vi "PS Control (RT).vi"() -> ()   [LabVIEW 2019]
uses:
  <vilib>/rvi/interface/nirviReadWriteControl/nirviReadWriteControl.xnode
  <vilib>/rvi/interface/Simulation/niFpgaSimulationCallBeginRW.vi
  <vilib>/rvi/errors/niLvFpgaAdjustHostInterfaceError.vi
  <vilib>/addons/control/pid/NI_PID_pid.lvlib
  <vilib>/addons/control/pid/pid.llb/PID (DBL).vi
  <vilib>/rvi/interface/nirviOpenFPGA/nirviOpenFPGA.xnode
  FPGA/bitfiles/PS Control (FPGA).lvbitx
  <vilib>/ptbypt/NI_PtbyPt.lvlib
  <vilib>/Analysis/3filter.llb/Filter Passband Type.ctl
  <vilib>/Analysis/NI_AALBase.lvlib
  <vilib>/FPGAPlugInAG/sbRIO-9626/niLvFpga_Open_sbRIO-9626.vi
  <vilib>/rvi/interface/common/dynamic/niFpgaDynamicAddResources.vi
panel:
  in  "PS4 Remote Control":bool=TRUE
  in  "PS3 Remote Control":bool=TRUE
  in  "PS2 Remote Control":bool=TRUE
  in  "PS1 Remote Control":bool=TRUE
  out "CPU Usage:":dbl=7.74131899555212 format="%.1f"
  in  "Scale 4":dbl=2.0
  in  "Offset 4":dbl
  out "AI 3":fxp<+/-,24,5>
  in  "PS CMD 4":dbl format="%.2f"
  in  "dt (s) 4":dbl=-1.0 format="%.3f"
  in  "PID gains 4":T1={"proportional gain"=1.0, "integral time"=0.01, "derivative time"=0.0} {"derivative time" format="%.3f"; "integral time" format="%.3f"; "proportional gain" format="%.3f"}
  in  "Output Range 4":cluster{"output high":dbl, "output low":dbl}={"output high"=8.0, "output low"=0.0} {"output low" format="%.2f"; "output high" format="%.2f"}
  out "PS Feedback 4":dbl format="%0.2f"
  out "AO 3":fxp<+/-,20,5>
  in  "Scale 3":dbl=2.0
  in  "Offset 3":dbl
  out "AI 2":fxp<+/-,24,5>
  in  "PS CMD 3":dbl format="%.2f"
  in  "dt (s) 3":dbl=-1.0 format="%.3f"
  in  "PID gains 3":T1={"proportional gain"=1.0, "integral time"=0.01, "derivative time"=0.0} {"derivative time" format="%.3f"; "integral time" format="%.3f"; "proportional gain" format="%.3f"}
  in  "Output Range 3":cluster{"output high":dbl, "output low":dbl}={"output high"=8.0, "output low"=0.0} {"output low" format="%.2f"; "output high" format="%.2f"}
  out "PS Feedback 3":dbl format="%0.2f"
  out "AO 2":fxp<+/-,20,5>
  in  "Scale 2":dbl=2.0
  in  "Offset 2":dbl
  out "AI 1":fxp<+/-,24,5>
  in  "PS CMD 2":dbl format="%.2f"
  in  "dt (s) 2":dbl=-1.0 format="%.3f"
  in  "PID gains 2":T1={"proportional gain"=1.0, "integral time"=0.01, "derivative time"=0.0} {"derivative time" format="%.3f"; "integral time" format="%.3f"; "proportional gain" format="%.3f"}
  in  "Output Range 2":cluster{"output high":dbl, "output low":dbl}={"output high"=8.0, "output low"=0.0} {"output low" format="%.2f"; "output high" format="%.2f"}
  out "PS Feedback 2":dbl format="%0.2f"
  out "AO 1":fxp<+/-,20,5>
  in  "Loop Timer (uSec)":u32=10000
  out "AO 0":fxp<+/-,20,5>
  out "PS Feedback 1":dbl format="%0.2f"
  in  "Output Range 1":cluster{"output high":dbl, "output low":dbl}={"output high"=8.0, "output low"=0.0} {"output low" format="%.2f"; "output high" format="%.2f"}
  in  "PID gains 1":T1={"proportional gain"=1.0, "integral time"=0.01, "derivative time"=0.0} {"derivative time" format="%.3f"; "integral time" format="%.3f"; "proportional gain" format="%.3f"}
  in  "dt (s) 1":dbl=-1.0 format="%.3f"
  in  "PS CMD 1":dbl format="%.2f"
  out "AI 0":fxp<+/-,24,5>
  in  "Offset":dbl
  in  "Scale":dbl=2.0
  # "Power Supply 1"
  # "Power Supply 2"
  # "Power Supply 3"
  # "Power Supply 4"
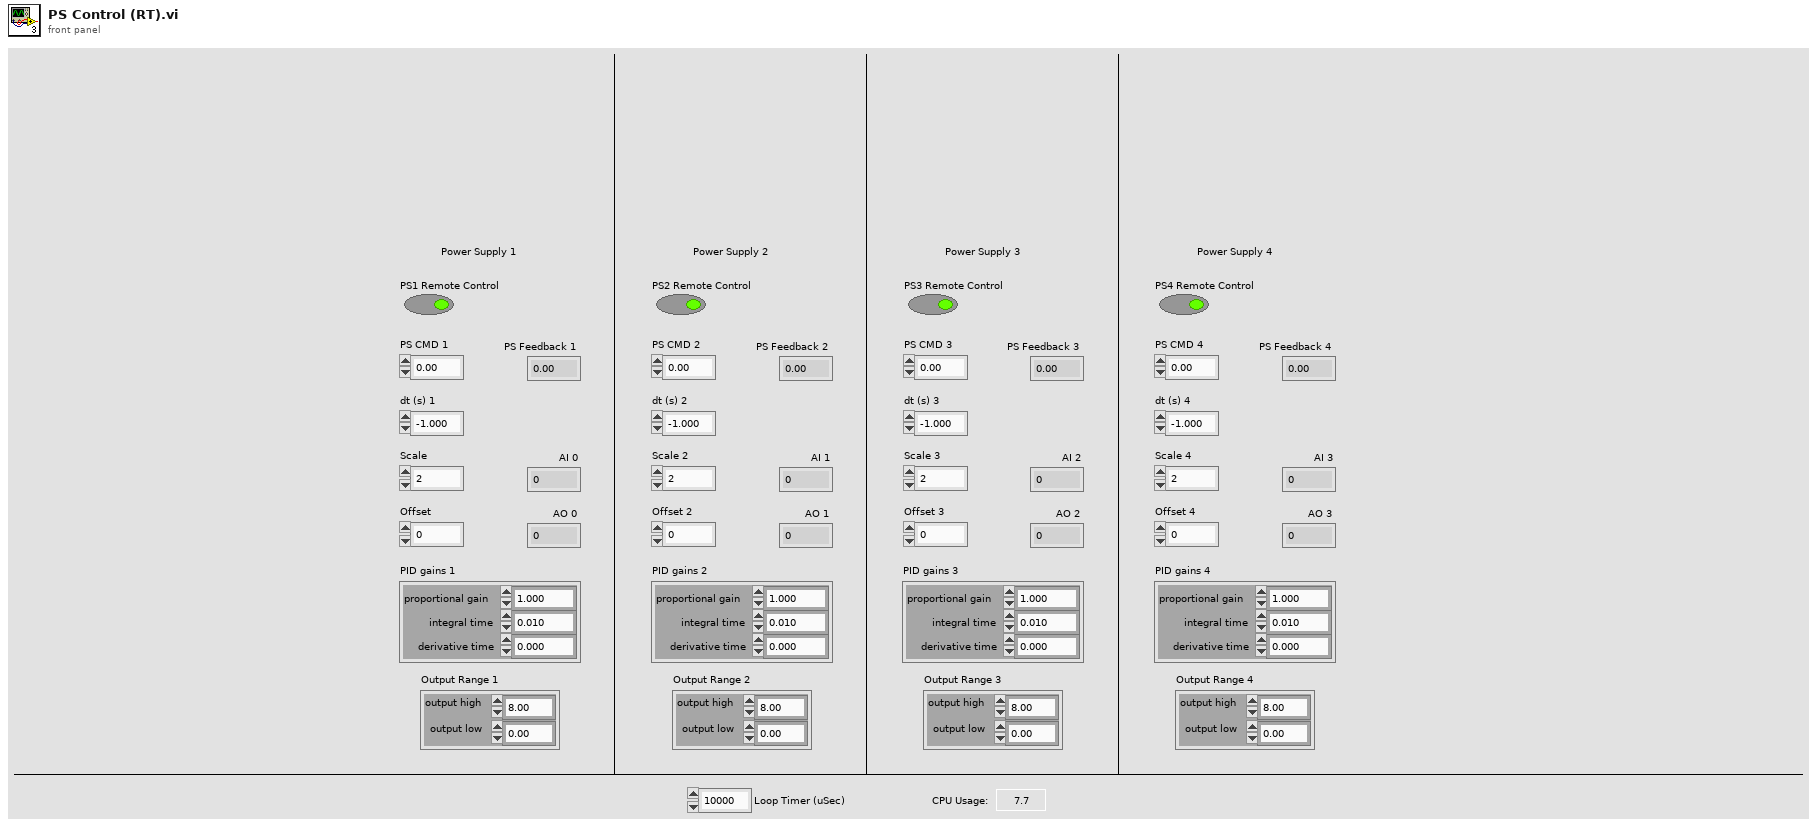
[diagram p1: front panel]
types:
  T1 = cluster{"proportional gain":dbl, "integral time":dbl, "derivative time":dbl}
  T2 = typedef "NI_AALBase.lvlib/Filter Passband Type.ctl" = enum32{"Lowpass", "Highpass", "Bandpass", "Bandstop"}
  T3 = typedef "NI_Real-Time Target Support.lvlib/RT CPU Load.ctl" = cluster{"Total (%)":dbl, "Time Critical (%)":dbl, "Timed Structures (%)":dbl, "High (%)":dbl, "Above Normal (%)":dbl, "Normal (%)":dbl, "Background (%)":dbl, "Idle (%)":dbl, "ISR (%)":dbl}
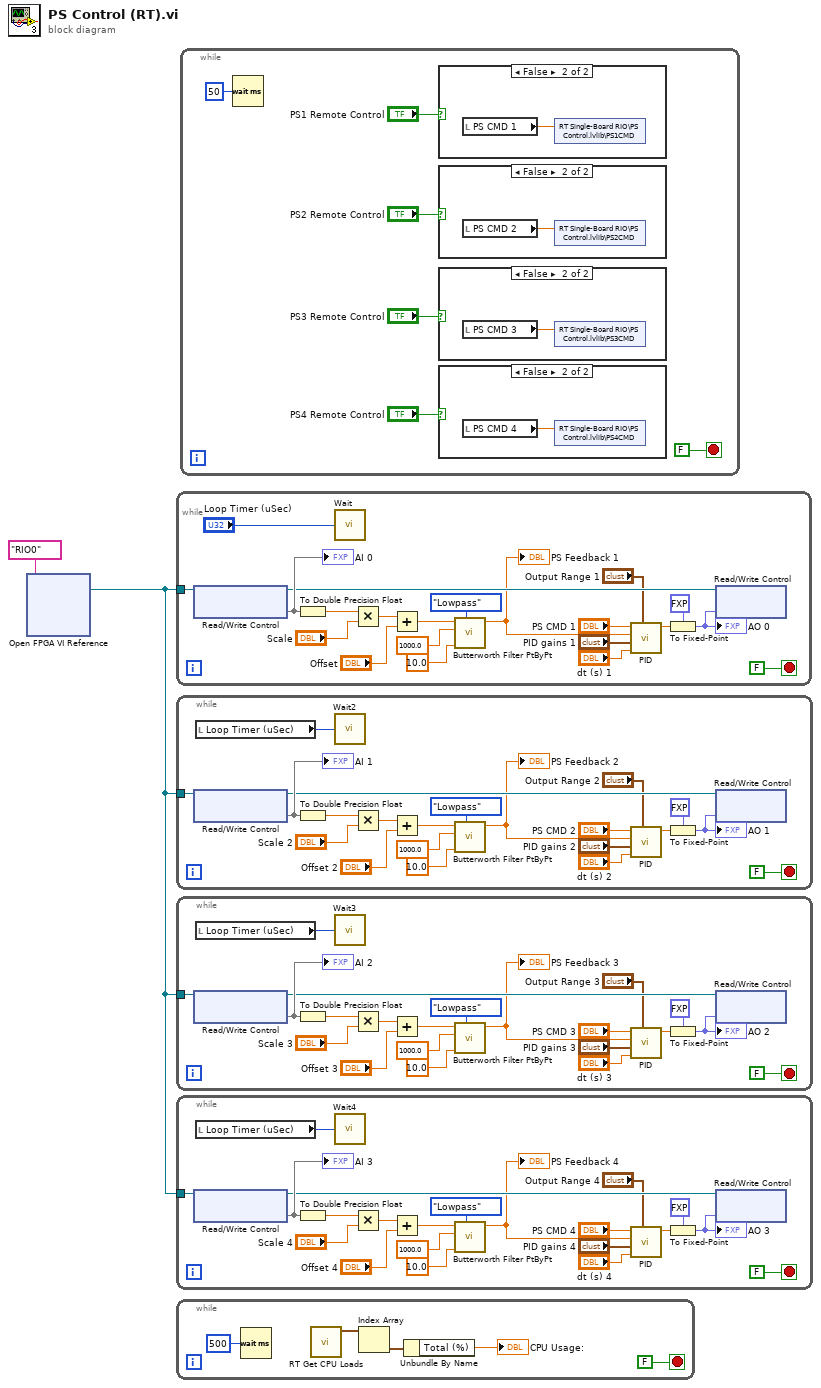
[diagram p0: block diagram]
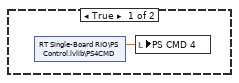
[diagram p2: hidden frame]
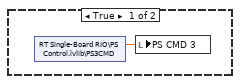
[diagram p3: hidden frame]
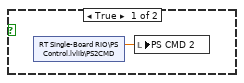
[diagram p4: hidden frame]
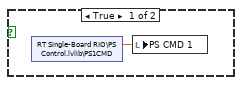
[diagram p5: hidden frame]
diagram:
  n1 = xnode "Open FPGA VI Reference"("resource name"=tag "RIO0") -> ("FPGA VI Reference Out"=w1:refnum<k20>)  [unwired: 1 in, 1 out]
  n2 = while {
    tunnel: w1 -> [w18]
    stop <- FALSE stop-if-true
    n3 = xnode "Read/Write Control"("FPGA VI Reference In"=w18) -> ("FPGA VI Reference Out"=w17:refnum<k20>, "PS Feedback 1"=w21)  [unwired: 1 in, 1 out]
    "AI 0" <- w21
    n4 = To Double Precision Float(number=w21) -> (double precision float=w20:dbl)
    n5 = call "Wait"("Count(uSec)"="Loop Timer (uSec)") -> ()  [unwired: 1 out]
    n6 = Multiply(x=w20, y="Scale") -> (x*y=w19:dbl)
    n7 = Add(x=w19, y="Offset") -> (x+y=w11:dbl)
    n8 = call <vilib>:"Butterworth Filter PtByPt.vi"("filter type"=Filter_Passband_Type."Lowpass", "low cutoff freq: fl"=10.0, "sampling freq: fs"=1000.0, "x"=w11) -> ("Filtered x"=w7:dbl)  [unwired: 5 in, 1 out]
    "PS Feedback 1" <- w7
    n9 = call-poly <vilib>:"PID.vi"("output range"="Output Range 1", "dt (s)"="dt (s) 1", "PID gains"="PID gains 1", "process variable"=w7, "setpoint"="PS CMD 1") -> ("output"=w4:dbl)  [unwired: 5 in, 1 out]
    n10 = To Fixed-Point(fixed-point type=fxp<+/-,20,5> 0.0 ("PS CMD 1"), number=w4) -> (fixed-point=w3:fxp<+/-,20,5>)
    "AO 0" <- w3
    n11 = xnode "Read/Write Control"("FPGA VI Reference In"=w17, "PS CMD 1"=w3) -> ()  [unwired: 1 in, 2 out]
  }
  n12 = while {
    tunnel: w1 -> [w39]
    stop <- FALSE stop-if-true
    n13 = xnode "Read/Write Control"("FPGA VI Reference In"=w39) -> ("FPGA VI Reference Out"=w38:refnum<k20>, "PS Feedback 2"=w42)  [unwired: 1 in, 1 out]
    "AI 1" <- w42
    n14 = local read "Loop Timer (uSec)"() -> (w27:u32)
    n15 = To Double Precision Float(number=w42) -> (double precision float=w41:dbl)
    n16 = call "Wait2"("Count(uSec)"=w27) -> ()  [unwired: 1 out]
    n17 = Multiply(x=w41, y="Scale 2") -> (x*y=w40:dbl)
    n18 = Add(x=w40, y="Offset 2") -> (x+y=w32:dbl)
    n19 = call <vilib>:"Butterworth Filter PtByPt.vi"("filter type"=Filter_Passband_Type."Lowpass", "low cutoff freq: fl"=10.0, "sampling freq: fs"=1000.0, "x"=w32) -> ("Filtered x"=w28:dbl)  [unwired: 5 in, 1 out]
    "PS Feedback 2" <- w28
    n20 = call-poly <vilib>:"PID.vi"("output range"="Output Range 2", "dt (s)"="dt (s) 2", "PID gains"="PID gains 2", "process variable"=w28, "setpoint"="PS CMD 2") -> ("output"=w24:dbl)  [unwired: 5 in, 1 out]
    n21 = To Fixed-Point(fixed-point type=fxp<+/-,20,5> 0.0 ("PS CMD 1"), number=w24) -> (fixed-point=w26:fxp<+/-,20,5>)
    "AO 1" <- w26
    n22 = xnode "Read/Write Control"("FPGA VI Reference In"=w38, "PS CMD 2"=w26) -> ()  [unwired: 1 in, 2 out]
  }
  n23 = while {
    tunnel: w1 -> [w60]
    stop <- FALSE stop-if-true
    n24 = xnode "Read/Write Control"("FPGA VI Reference In"=w60) -> ("FPGA VI Reference Out"=w59:refnum<k20>, "PS Feedback 3"=w63)  [unwired: 1 in, 1 out]
    "AI 2" <- w63
    n25 = local read "Loop Timer (uSec)"() -> (w48:u32)
    n26 = To Double Precision Float(number=w63) -> (double precision float=w62:dbl)
    n27 = call "Wait3"("Count(uSec)"=w48) -> ()  [unwired: 1 out]
    n28 = Multiply(x=w62, y="Scale 3") -> (x*y=w61:dbl)
    n29 = Add(x=w61, y="Offset 3") -> (x+y=w53:dbl)
    n30 = call <vilib>:"Butterworth Filter PtByPt.vi"("filter type"=Filter_Passband_Type."Lowpass", "low cutoff freq: fl"=10.0, "sampling freq: fs"=1000.0, "x"=w53) -> ("Filtered x"=w49:dbl)  [unwired: 5 in, 1 out]
    "PS Feedback 3" <- w49
    n31 = call-poly <vilib>:"PID.vi"("output range"="Output Range 3", "dt (s)"="dt (s) 3", "PID gains"="PID gains 3", "process variable"=w49, "setpoint"="PS CMD 3") -> ("output"=w45:dbl)  [unwired: 5 in, 1 out]
    n32 = To Fixed-Point(fixed-point type=fxp<+/-,20,5> 0.0 ("PS CMD 1"), number=w45) -> (fixed-point=w47:fxp<+/-,20,5>)
    "AO 2" <- w47
    n33 = xnode "Read/Write Control"("FPGA VI Reference In"=w59, "PS CMD 3"=w47) -> ()  [unwired: 1 in, 2 out]
  }
  n34 = while {
    tunnel: w1 -> [w81]
    stop <- FALSE stop-if-true
    n35 = xnode "Read/Write Control"("FPGA VI Reference In"=w81) -> ("FPGA VI Reference Out"=w80:refnum<k20>, "PS Feedback 4"=w84)  [unwired: 1 in, 1 out]
    "AI 3" <- w84
    n36 = local read "Loop Timer (uSec)"() -> (w69:u32)
    n37 = To Double Precision Float(number=w84) -> (double precision float=w83:dbl)
    n38 = call "Wait4"("Count(uSec)"=w69) -> ()  [unwired: 1 out]
    n39 = Multiply(x=w83, y="Scale 4") -> (x*y=w82:dbl)
    n40 = Add(x=w82, y="Offset 4") -> (x+y=w74:dbl)
    n41 = call <vilib>:"Butterworth Filter PtByPt.vi"("filter type"=Filter_Passband_Type."Lowpass", "low cutoff freq: fl"=10.0, "sampling freq: fs"=1000.0, "x"=w74) -> ("Filtered x"=w70:dbl)  [unwired: 5 in, 1 out]
    "PS Feedback 4" <- w70
    n42 = call-poly <vilib>:"PID.vi"("output range"="Output Range 4", "dt (s)"="dt (s) 4", "PID gains"="PID gains 4", "process variable"=w70, "setpoint"="PS CMD 4") -> ("output"=w66:dbl)  [unwired: 5 in, 1 out]
    n43 = To Fixed-Point(fixed-point type=fxp<+/-,20,5> 0.0 ("PS CMD 1"), number=w66) -> (fixed-point=w68:fxp<+/-,20,5>)
    "AO 3" <- w68
    n44 = xnode "Read/Write Control"("FPGA VI Reference In"=w80, "PS CMD 4"=w68) -> ()  [unwired: 1 in, 2 out]
  }
  n45 = while {
    stop <- FALSE stop-if-true
    n46 = Wait (ms)(milliseconds to wait=u32 500) -> ()  [unwired: 1 out]
    n47 = call <vilib>:"RT Get CPU Loads.vi"() -> ("CPU loads"=w89:T3[])  [unwired: 10 in, 1 out]
    n48 = Index Array(array=w89) -> (element=w90:T3)  [unwired: 1 in]
    n49 = Unbundle By Name(w90) -> ("Total (%)"=→"CPU Usage:":dbl)
  }
  n50 = while {
    stop <- FALSE stop-if-true
    n51 = Wait (ms)(milliseconds to wait=u32 50) -> ()  [unwired: 1 out]
    n52 = case shown="False" "PS1 Remote Control" {
      frame True {
        n53 = shared-variable "RT Single-Board RIO\\PS Control.lvlib\\PS1CMD"() -> (w104:dbl)  [unwired: 1 in, 1 out]
        n54 = local write "PS CMD 1"(w104) -> ()
      }
      frame False {
        n55 = local read "PS CMD 1"() -> (w105:dbl)
        n56 = shared-variable "RT Single-Board RIO\\PS Control.lvlib\\PS1CMD"(w105) -> ()  [unwired: 1 in, 1 out]
      }
    }
    n57 = case shown="False" "PS2 Remote Control" {
      frame True {
        n58 = shared-variable "RT Single-Board RIO\\PS Control.lvlib\\PS2CMD"() -> (w102:dbl)  [unwired: 1 in, 1 out]
        n59 = local write "PS CMD 2"(w102) -> ()
      }
      frame False {
        n60 = local read "PS CMD 2"() -> (w103:dbl)
        n61 = shared-variable "RT Single-Board RIO\\PS Control.lvlib\\PS2CMD"(w103) -> ()  [unwired: 1 in, 1 out]
      }
    }
    n62 = case shown="False" "PS3 Remote Control" {
      frame True {
        n63 = shared-variable "RT Single-Board RIO\\PS Control.lvlib\\PS3CMD"() -> (w100:dbl)  [unwired: 1 in, 1 out]
        n64 = local write "PS CMD 3"(w100) -> ()
      }
      frame False {
        n65 = local read "PS CMD 3"() -> (w101:dbl)
        n66 = shared-variable "RT Single-Board RIO\\PS Control.lvlib\\PS3CMD"(w101) -> ()  [unwired: 1 in, 1 out]
      }
    }
    n67 = case shown="False" "PS4 Remote Control" {
      frame True {
        n68 = shared-variable "RT Single-Board RIO\\PS Control.lvlib\\PS4CMD"() -> (w98:dbl)  [unwired: 1 in, 1 out]
        n69 = local write "PS CMD 4"(w98) -> ()
      }
      frame False {
        n70 = local read "PS CMD 4"() -> (w99:dbl)
        n71 = shared-variable "RT Single-Board RIO\\PS Control.lvlib\\PS4CMD"(w99) -> ()  [unwired: 1 in, 1 out]
      }
    }
  }
